vi "tra.vi"() -> ()   [LabVIEW 2020]
uses:
  Database/Global1.vi
  <vilib>/addons/database/Connection.llb/DB Tools Open Connec (String).vi
  <vilib>/addons/database/Connection.llb/Conn Execute.vi
  <vilib>/addons/database/Recordset.llb/Rec Fetch Recordset Data (R).vi
  <vilib>/addons/database/NI_Database_API.lvlib
  <vilib>/addons/database/Connection.llb/DB Tools Open Connec (Path).vi
panel:
  out "字符串 2":string
  out "字符串":string
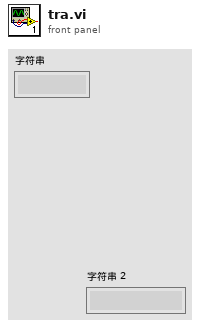
[diagram p1: front panel]
types:
  T1 = cluster{"长度":i64, "长度":i64, string, sgl, sgl, string, string, string}
  T2 = cluster{"长度":i64, "长度":i64, string, sgl, sgl, string, string, string}[]
  T3 = typedef "NI_Database_API.lvlib/Conn ObjectReference.ctl" = refnum<k1>
  T4 = cluster{"长度":i64, "长度":i64, sgl, sgl, string, string, string}
  T5 = typedef "NI_Database_API.lvlib/Rec ObjectReference.ctl" = refnum<k1>
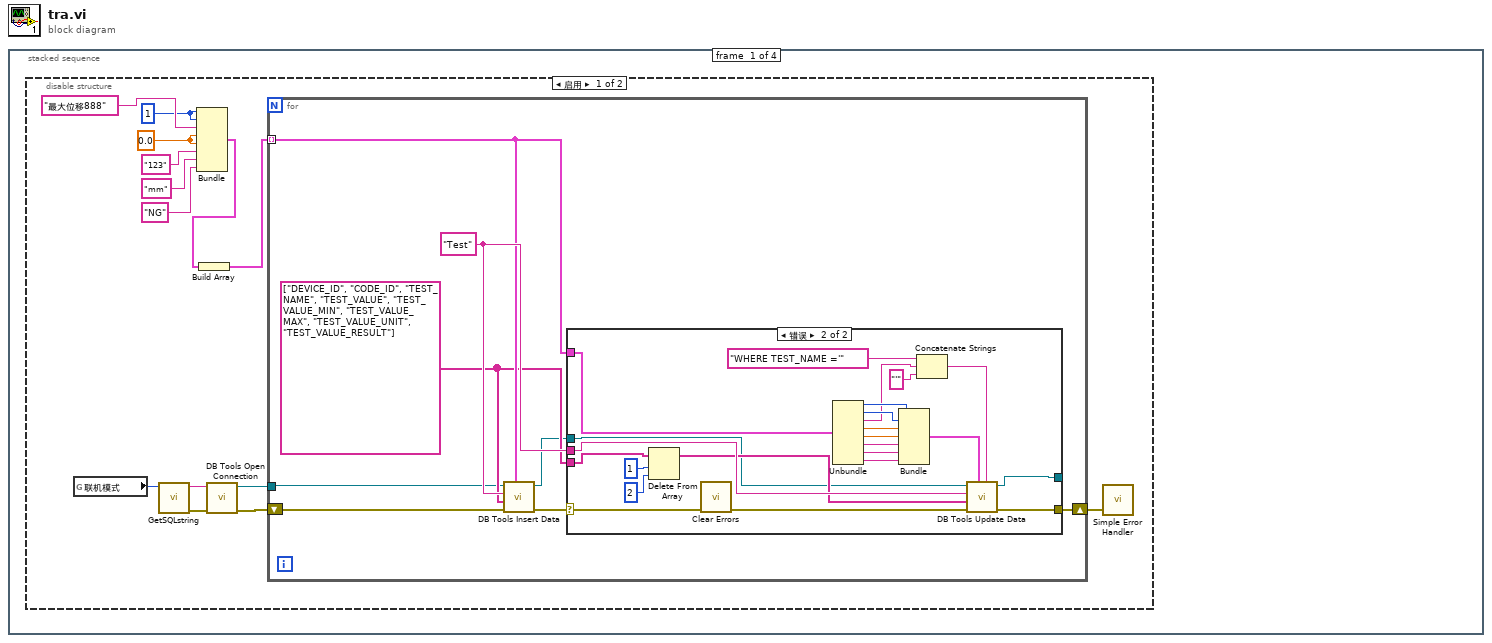
[diagram p0: block diagram]
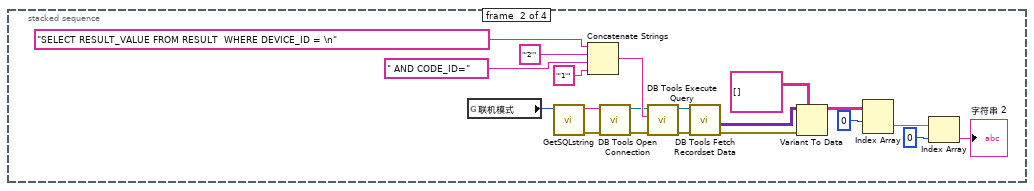
[diagram p4: hidden frame]
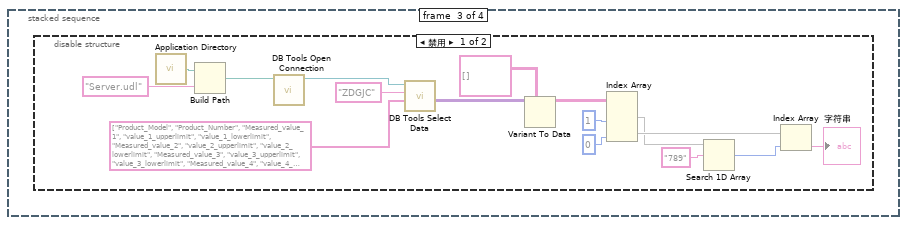
[diagram p5: hidden frame]
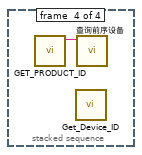
[diagram p7: hidden frame]
diagram:
  n1 = stacked-sequence {
    frame #0 {
      n2 = disable-structure shown="启用" {
        frame Enabled {
          w4 = sgl 0.0
          w5 = i64 1 ("长度")
          n3 = global read "Global1.vi" "联机模式"() -> (w13:enum16{"单机", "追溯"})
          n4 = call "GetSQLstring.vi"("联机模式"=w13) -> ("错误输出"=w11:errorcluster, "连接字符串"=w12:string)  [unwired: 9 in]
          n5 = Bundle("长度"=w5, "长度"=w5, "最大位移888", w4, w4, "123", "mm", "NG") -> (w2:T1)  [unwired: 1 in]
          n6 = Build Array(w2) -> (w1:T2)
          n7 = call-poly <vilib>:"DB Tools Open Connection.vi"("error in (no error)"=w11, "connection information"=w12) -> ("error out"=w14:errorcluster, "connection reference"=w8:T3)  [unwired: 6 in]
          n8 = for {
            tunnel: w1 -> [w19] mode=indexing
            tunnel: w8 -> [w17]
            shift-right: [w15] -> w3
            shift-left: w14 -> [w22]
            w18 = string[] ["DEVICE_ID", "CODE_ID", "TEST_NAME", "TEST_VALUE", "TEST_VALUE_MIN", "TEST_VALUE_MAX", "TEST_VALUE_UNIT", "TEST_VALUE_RESULT"] ("columns")
            w20 = "Test" ("table")
            n9 = call <vilib>:"DB Tools Insert Data.vi"("data"=w19, "error in (no error)"=w22, "columns"=w18, "table"=w20, "connection reference"=w17) -> ("error out"=w21:errorcluster, "connection reference out"=w16:T3)  [unwired: 5 in]
            n10 = case shown="错误" w21 {
              selector: w21 -> [w23 w46]
              tunnel: w18 -> [_ w43]
              tunnel: w16 -> [w24 w27]
              tunnel: w20 -> [_ w47]
              tunnel: w19 -> [_ w37]
              tunnel: [w24 w26] -> _
              tunnel: [w23 w25] -> w15
              frame No Error {
              }
              frame Error {
                n11 = Delete From Array(array=w43, length=1 ("长度"), index=2 ("索引")) -> (array with subset deleted=w44:string[])  [unwired: 1 out]
                n12 = call <vilib>:"Clear Errors.vi"("error in (no error)"=w46) -> ("error out"=w45:errorcluster)  [unwired: 5 in, 1 out]
                n13 = Unbundle(w37) -> ("长度"=w36:i64, "长度"=w35:i64, w28:string, w34:sgl, w33:sgl, w32:string, w31:string, w30:string)
                n14 = Bundle("长度"=w36, "长度"=w35, w34, w33, w32, w31, w30) -> (w29:T4)  [unwired: 1 in]
                n15 = Concatenate Strings("WHERE TEST_NAME ='" ("condition"), w28, "'") -> (w39:string)
                n16 = call <vilib>:"DB Tools Update Data.vi"("condition"=w39, "data"=w29, "error in (no error)"=w45, "columns"=w44, "table"=w47, "connection reference"=w27) -> ("error out"=w25:errorcluster, "connection reference out"=w26:T3)  [unwired: 4 in]
              }
            }
          }
          n17 = call <vilib>:"Simple Error Handler.vi"("error in (no error)"=w3) -> ()  [unwired: 4 in, 5 out]
        }
        frame Disabled {
        }
      }
    }
    frame #1 {
      n18 = global read "Global1.vi" "联机模式"() -> (w67:enum16{"单机", "追溯"})
      n19 = call "GetSQLstring.vi"("联机模式"=w67) -> ("错误输出"=w65:errorcluster, "连接字符串"=w66:string)  [unwired: 9 in]
      n20 = Concatenate Strings("SELECT RESULT_VALUE FROM RESULT  WHERE DEVICE_ID = \n" ("table"), "'2'" ("字符串"), " AND CODE_ID=" ("字符串"), "'1'" ("字符串")) -> (w64:string)
      n21 = call-poly <vilib>:"DB Tools Open Connection.vi"("error in (no error)"=w65, "connection information"=w66) -> ("error out"=w58:errorcluster, "connection reference"=w59:T3)  [unwired: 6 in]
      n22 = call-poly <vilib>:"DB Tools Execute Query.vi"("error in (no error)"=w58, "SQL query"=w64, "connection reference"=w59) -> ("error out"=w62:errorcluster, "recordset reference"=w63:T5)  [unwired: 5 in]
      n23 = call-poly <vilib>:"DB Tools Fetch Recordset Data.vi"("error in (no error)"=w62, "recordset reference"=w63) -> ("error out"=w53:errorcluster, "recordset data"=w61:variant[][])  [unwired: 3 in, 1 out]
      n24 = Variant To Data(error in=w53, type=string[][] [], Variant=w61) -> (data=w52:string[][])  [unwired: 1 out]
      n25 = Index Array(array=w52, index (row)=0 ("索引 (行)")) -> (element=w50:string[])  [unwired: 1 in]
      n26 = Index Array(array=w50, index=0 ("索引")) -> (element=→"字符串 2":string)
    }
    frame #2 {
      n27 = disable-structure shown="禁用" {
        frame Disabled {
          n28 = call <vilib>:"Application Directory.vi"() -> ("Application Directory"=w79:path)
          n29 = Build Path(base path=w79, name or relative path="Server.udl") -> (appended path=w78:path)
          n30 = call-poly <vilib>:"DB Tools Open Connection.vi"("connection information"=w78) -> ("connection reference"=w77:T3)  [unwired: 7 in, 1 out]
          n31 = call <vilib>:"DB Tools Select Data.vi"("columns"=string[] ["Product_Model", "Product_Number", "Measured_value_1", "value_1_upperlimit", "value_1_lowerlimit", "Measured_value_2", "value_2_upperlimit", "value_2_lowerlimit", "Measured_value_3", "value_3_upperlimit", "value_3_lowerlimit", "Measured_value_4", "value_4_upperlimit", "value_4_lowerlimit", "Measured_value_5", "value_5_upperlimit", "value_5_lowerlimit", "Measured_value_6", "value_6_upperlimit", "value_6_lowerlimit", "Measured_value_7", "value_7_upperlimit", "value_7_lowerlimit", "Measured_value_8", "value_8_upperlimit", "value_8_lowerlimit", "Measured_value_9", "value_9_upperlimit", "value_9_lowerlimit", "Measured_value_10", "value_10_upperlimit", "value_10_lowerlimit"], "table"="ZDGJC", "connection reference"=w77) -> ("data"=w76:variant[][])  [unwired: 3 in, 2 out]
          n32 = Variant To Data(type=string[][] [], Variant=w76) -> (data=w74:string[][])  [unwired: 1 in, 1 out]
          n33 = Index Array(array=w74, index (col) #1=1 ("禁用的索引 (列)"), index (col) #2=0 ("索引 (列)")) -> (element #1=w70:string[], element #2=w71:string[])  [unwired: 2 in]
          n34 = Search 1D Array(1D array=w70, element="789" ("元素")) -> (index of element=w81:i32)  [unwired: 1 in]
          n35 = Index Array(array=w71, index=w81) -> (element=→"字符串":string)
        }
        frame Enabled {
        }
      }
    }
    frame #3 {
      n36 = call "GET_PRODUCT_ID.vi"() -> ("PRODUCT_ID"=w84:string)  [unwired: 11 in]
      n37 = call "Get_Device_ID.vi"() -> ()  [unwired: 10 in, 2 out]
      n38 = call "查询前序设备.vi"("PRODUCT_ID"=w84) -> ()  [unwired: 10 in, 1 out]
    }
  }
